vi "Execute Msg.vi"(7 "Actor in":refnum<class "Actor.lvclass">, 8 "Error in":errorcluster, 11 "Stopped Msg in":refnum<class "Stopped Msg.lvclass">) -> (0 "Error out":errorcluster, 2 "Msg Output":refnum<class "Msg Output.lvclass">, 5 "Actor out":refnum<class "Actor.lvclass">)   [LabVIEW 2025, in "jettl.lvlib" / "Stopped jettl Msg.lvlib" / "Stopped Msg.lvlib" / "Stopped Msg.lvclass"]
uses:
  Stopped Msg.lvclass
  Stopped Msg.lvclass/Stopped Msg.ctl
  Stopped jettl Msg/Stopped jettl Msg.lvclass
  Actor/Actor.lvclass
  Msg Output/Msg Output.lvclass
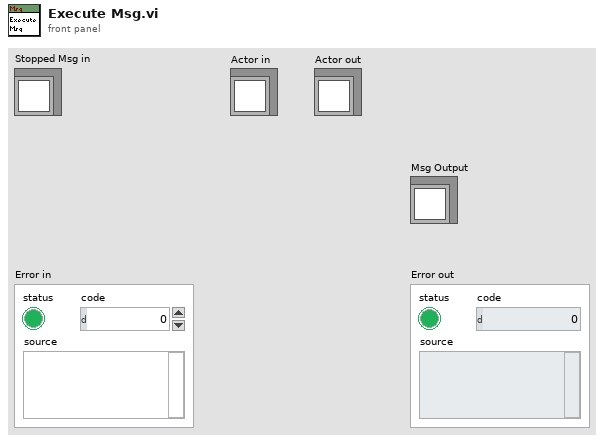
[diagram p1: front panel]
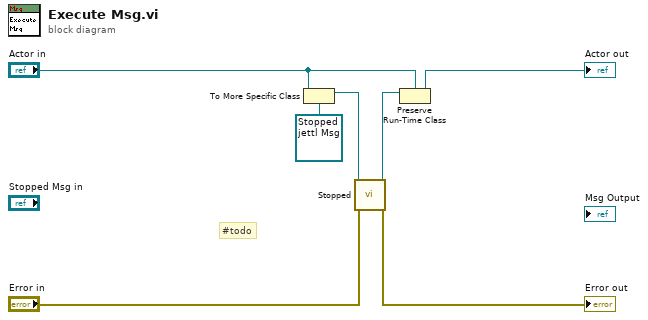
[diagram p0: block diagram]
diagram:
  # "#todo"
  n1 = To More Specific Class(target class=refnum<class "Stopped jettl Msg.lvclass"> refnum ("jettl.lvlib:jettl Msg Last Ack Creator Queue.lvlib:jettl Msg Last Ack Creator Queue.lvclass"), reference="Actor in") -> (specific class reference=w2:refnum<class "Stopped jettl Msg.lvclass">)  [unwired: 1 in, 1 out]
  n2 = call-dynamic "Stopped.vi"("Error in"="Error in", "Stopped jettl Msg in"=w2) -> ("Error out"=→"Error out":errorcluster, "Stopped jettl Msg out"=w1:refnum<class "Stopped jettl Msg.lvclass">)  [unwired: 8 in]
  n3 = Preserve Run-Time Class(object in=w1, 2:"Actor in") -> (object out=→"Actor out":refnum<class "Actor.lvclass">)  [unwired: 1 in, 1 out]
